vi "callback_recv.vi"(8 "error in (no error)":errorcluster, 9 "flags":i32, 10 "length":u64, 11 "socket":u64) -> (0 "error out":errorcluster, 1 "buffer":u8[](array[numeric]), 2 "bytes received":i64)   [LabVIEW 2017, in "support.lvlib"]
doc: "Called when libssh2 wants to read data from the connection.\n\n<B>socket</B> the socket to read from.\n<B>length</B> number of bytes to read from the connection.\n<B>flags</B> flags that would have been used by a send() call.\n\nReturns the actual number of bytes received and the received bytes."
uses:
  support.lvlib
  ws2_32.dll
  libc.so.6
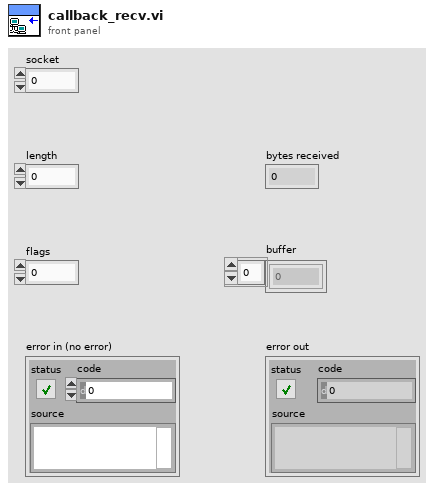
[diagram p1: front panel]
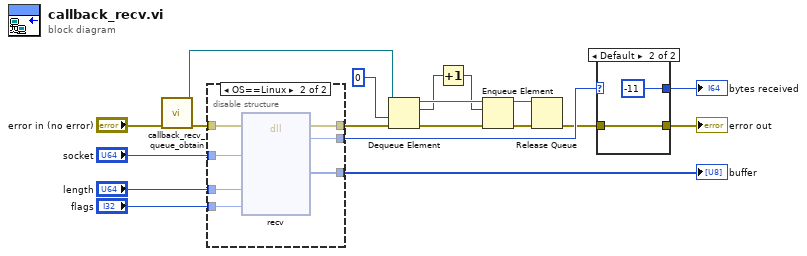
[diagram p0: block diagram]
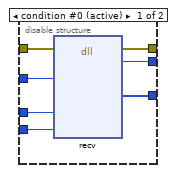
[diagram p2: hidden frame]
diagram:
  n1 = call "callback_recv_queue_obtain.vi"("error in (no error)"="error in (no error)") -> ("error out"=w12:errorcluster, "queue out"=w10:refnum<queue>)  [unwired: 9 in]
  n2 = disable-structure shown="OS==Linux" {
    disable-tunnel: "socket" -> [w26 w33]
    disable-tunnel: "length" -> [w25 w32]
    disable-tunnel: "flags" -> [w24 w31]
    disable-tunnel: [w23 w30] -> w15
    disable-tunnel: [w22 w29] -> w14
    disable-tunnel: w12 -> [w21 w28]
    disable-tunnel: [w20 w27] -> w9
    frame condition #0 (active) {
      n3 = dll-call lib="ws2_32.dll" fn="recv"(error in=w21, "s"=w26, "len"=w25, "flags"=w24) -> (error out=w22:errorcluster, "return type"=w20:i32, "buf"=w23:u8[])  [unwired: 6 in, 1 out]
    }
    frame condition #1 {
      n4 = dll-call lib="libc.so.6" fn="recv"(error in=w28, "sockfd"=w33, "size"=w32, "flags"=w31) -> (error out=w29:errorcluster, "return type"=w27:i32, "buf"=w30:u8[])  [unwired: 6 in, 1 out]
    }
  }
  "buffer" <- w15
  n5 = Dequeue Element(queue=w10, timeout in ms (-1)=0, error in (no error)=w14) -> (queue out=w5:refnum<queue>, element=w4:i32, error out=w11:errorcluster)  [unwired: 1 out]
  n6 = Increment(x=w4) -> (x+1=w3:i32)
  n7 = Enqueue Element(queue=w5, element=w3, error in (no error)=w11) -> (queue out=w6:refnum<queue>, error out=w7:errorcluster)  [unwired: 1 in, 1 out]
  n8 = Release Queue(queue=w6, error in (no error)=w7) -> (error out=w8:errorcluster)  [unwired: 1 in, 2 out]
  n9 = case shown="Default" w9 {
    selector: w9 -> [w35 _]
    tunnel: w8 -> [w34 w37]
    tunnel: [w34 w37] -> w13
    tunnel: [w35 -11] -> w1
    frame 0.. {
    }
    frame Default {
    }
  }
  "error out" <- w13
  "bytes received" <- w1
